vi "lookfordata_dbl.vi"(5 "Header":string, 6 "string (in)":string) -> (1 "output_string":string, 2 "output_dbl":dbl)   [LabVIEW 8.6]
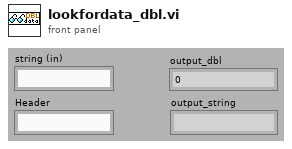
[diagram p1: front panel]
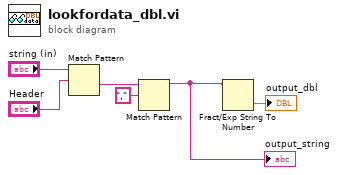
[diagram p0: block diagram]
diagram:
  n1 = Match Pattern(string="string (in)", regular expression="Header") -> (after substring=w3:string)  [unwired: 4 out]
  n2 = Match Pattern(string=w3, regular expression=",") -> (before substring=w2:string)  [unwired: 4 out]
  "output_string" <- w2
  n3 = Fract/Exp String To Number(string=w2) -> (number=→"output_dbl":dbl)  [unwired: 3 in, 1 out]
